vi "Subscribe.vi"(8 "error in (no error)":errorcluster, 9 "Multicast Port":u16, 10 "Multicast Address":string, 11 "RemoteDataService in":refnum<class "RemoteDataService.lvclass">) -> (0 "error out":errorcluster, 3 "RemoteDataService out":refnum<class "RemoteDataService.lvclass">)   [LabVIEW 2020, in "Vecto.lvlib" / "RemoteDataService.lvclass"]
uses:
  RemoteDataService.lvclass
  Subscribe Data.ctl
  Subscription.ctl
  RemoteDataService.lvclass/RemoteDataService.ctl
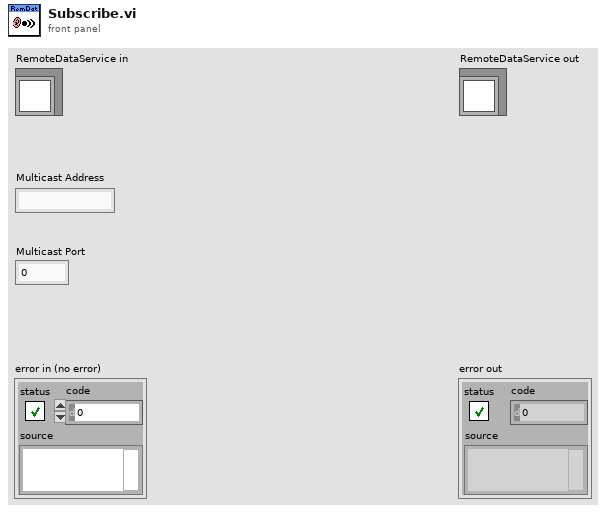
[diagram p1: front panel]
types:
  T1 = typedef "Vecto.lvlib/RemoteDataService.lvclass/Subscribe Data.ctl" = cluster{"Subscription":T2}
  T2 = typedef "Vecto.lvlib/RemoteDataService.lvclass/Subscription.ctl" = cluster{"Multicast Address":string, "Multicast Port":u16}
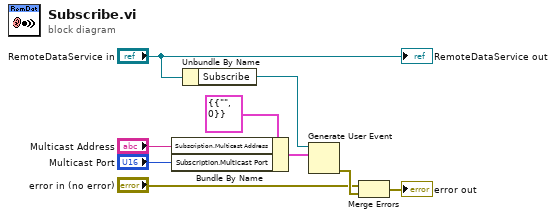
[diagram p0: block diagram]
diagram:
  n1 = Bundle By Name(cluster=T1 {"Subscription"={"Multicast Address"="", "Multicast Port"=0}} ("Subscribe Data"), "Subscription.Multicast Address"="Multicast Address", "Subscription.Multicast Port"="Multicast Port") -> (w5:T1)
  n2 = Unbundle By Name("RemoteDataService in") -> ("Subscribe"=w4:refnum<user-event>)
  n3 = Generate User Event(user event=w4, event data cluster=w5) -> (error out=w3:errorcluster)  [unwired: 2 in, 1 out]
  n4 = Merge Errors("error in (no error)", w3) -> (→"error out":errorcluster)
  "RemoteDataService out" <- "RemoteDataService in"
